vi "Main 硬體參數.vi"() -> ()   [LabVIEW 2015]
uses:
  <vilib>/Utility/miscctls.llb/LVPointTypeDef.ctl
panel:
  in  "切割刀數5":i32=10 min=0 max=10 step=1
  in  "功率5":i32=80 min=3 max=80 step=1
  in  "掃描速度5":i32=1000 min=0 max=10000 step=10
  out "output cluster":T1
  in  "?":T2={"掃描速度"=1000, "功率"=80, "切割刀數"=10, "角度"=10.0, "掃描速度2"=1000, "功率2"=80, "切割刀數2"=10, "角度2"=10.0, "掃描速度3"=1000, "功率3"=80, "切割刀數3"=10, "角度3"=10.0, "掃描速度4"=1000, "功率4"=80, "切割刀數4"=10, "角度4"=10.0, "左/右"=""} {"角度4" min=0.0 max=10.0 step=1.0; "角度3" min=0.0 max=10.0 step=1.0; "角度2" min=0.0 max=10.0 step=1.0; "角度" min=0.0 max=10.0 step=1.0; "切割刀數4" min=0 max=10 step=1; "功率4" min=3 max=80 step=1; "掃描速度4" min=0 max=1000 step=10; "切割刀數3" min=0 max=10 step=1; "功率3" min=3 max=80 step=1; "掃描速度3" min=0 max=1000 step=10; "切割刀數" min=0 max=10 step=1; "功率" min=3 max=80 step=1; "掃描速度" min=0 max=1000 step=10; "切割刀數2" max=10 step=1; "掃描速度2" min=0 max=1000 step=10; "功率2" min=3 max=80 step=1}
  in  "儲存":bool
  in  "離開":bool
  # "硬體參數"
  # "每日點檢"
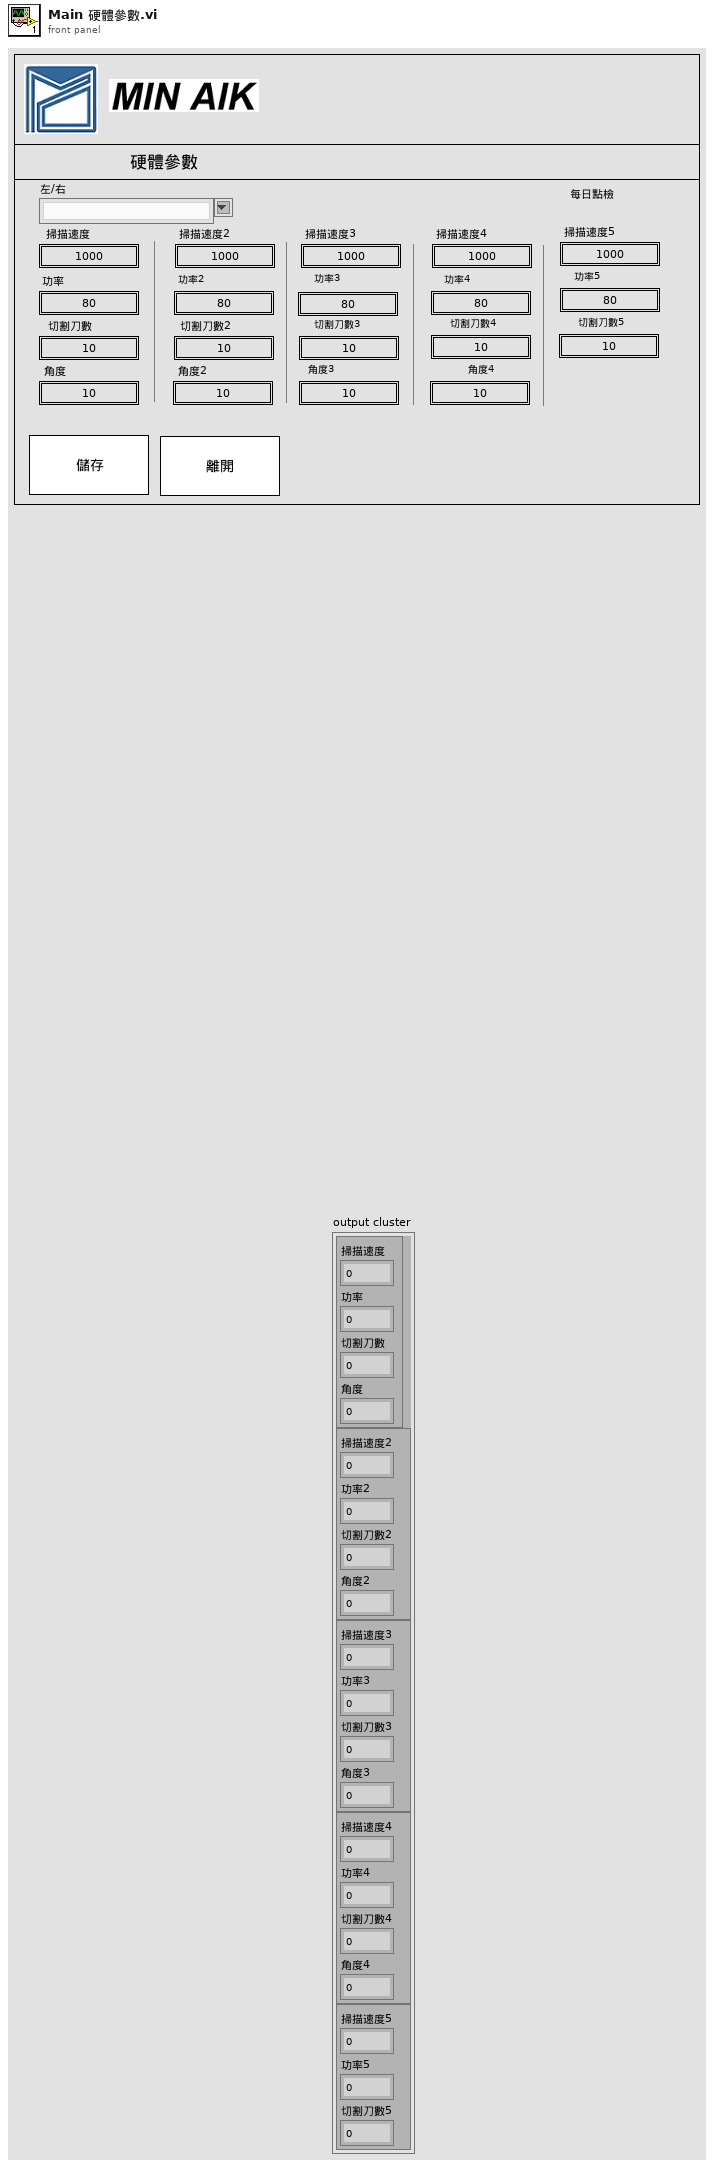
[diagram p1: front panel]
types:
  T1 = cluster{cluster{"掃描速度":i32, "功率":i32, "切割刀數":i32, "角度":dbl}, cluster{"掃描速度2":i32, "功率2":i32, "切割刀數2":i32, "角度2":dbl}, cluster{"掃描速度3":i32, "功率3":i32, "切割刀數3":i32, "角度3":dbl}, cluster{"掃描速度4":i32, "功率4":i32, "切割刀數4":i32, "角度4":dbl}, cluster{"掃描速度5":i32, "功率5":i32, "切割刀數5":i32}}
  T2 = cluster{"掃描速度":i32, "功率":i32, "切割刀數":i32, "角度":dbl, "掃描速度2":i32, "功率2":i32, "切割刀數2":i32, "角度2":dbl, "掃描速度3":i32, "功率3":i32, "切割刀數3":i32, "角度3":dbl, "掃描速度4":i32, "功率4":i32, "切割刀數4":i32, "角度4":dbl, "左/右":string}
  T3 = cluster{"功率":u8, "掃描速率(刀速) ":u16, "雷射半徑":dbl, "刀數":u32}
  T4 = typedef "Action_Data.ctl" = enum16{"Initialize", "Get Data", "Set Data", "Delete Data", "Idle"}
  T5 = typedef "LVPointTypeDef.ctl" = cluster{"Horizontal":i16, "Vertical":i16}
  T6 = cluster{"掃描速度":i32, "功率":i32, "切割刀數":i32, "角度":dbl}
  T7 = cluster{"掃描速度3":i32, "功率3":i32, "切割刀數3":i32, "角度3":dbl}
  T8 = cluster{"掃描速度4":i32, "功率4":i32, "切割刀數3":i32, "角度4":dbl}
  T9 = cluster{"掃描速度2":i32, "功率2":i32, "切割刀數":i32, "角度2":dbl}
  T10 = cluster{cluster{"掃描速度":i32, "功率":i32, "切割刀數":i32, "角度":dbl}, cluster{"掃描速度2":i32, "功率2":i32, "切割刀數":i32, "角度2":dbl}, cluster{"掃描速度3":i32, "功率3":i32, "切割刀數3":i32, "角度3":dbl}, cluster{"掃描速度4":i32, "功率4":i32, "切割刀數3":i32, "角度4":dbl}, cluster{"掃描速率(刀速) ":u16, "功率":u8, "刀數":u32}}
  T11 = cluster{"name or relative path":string, "Variant":variant}
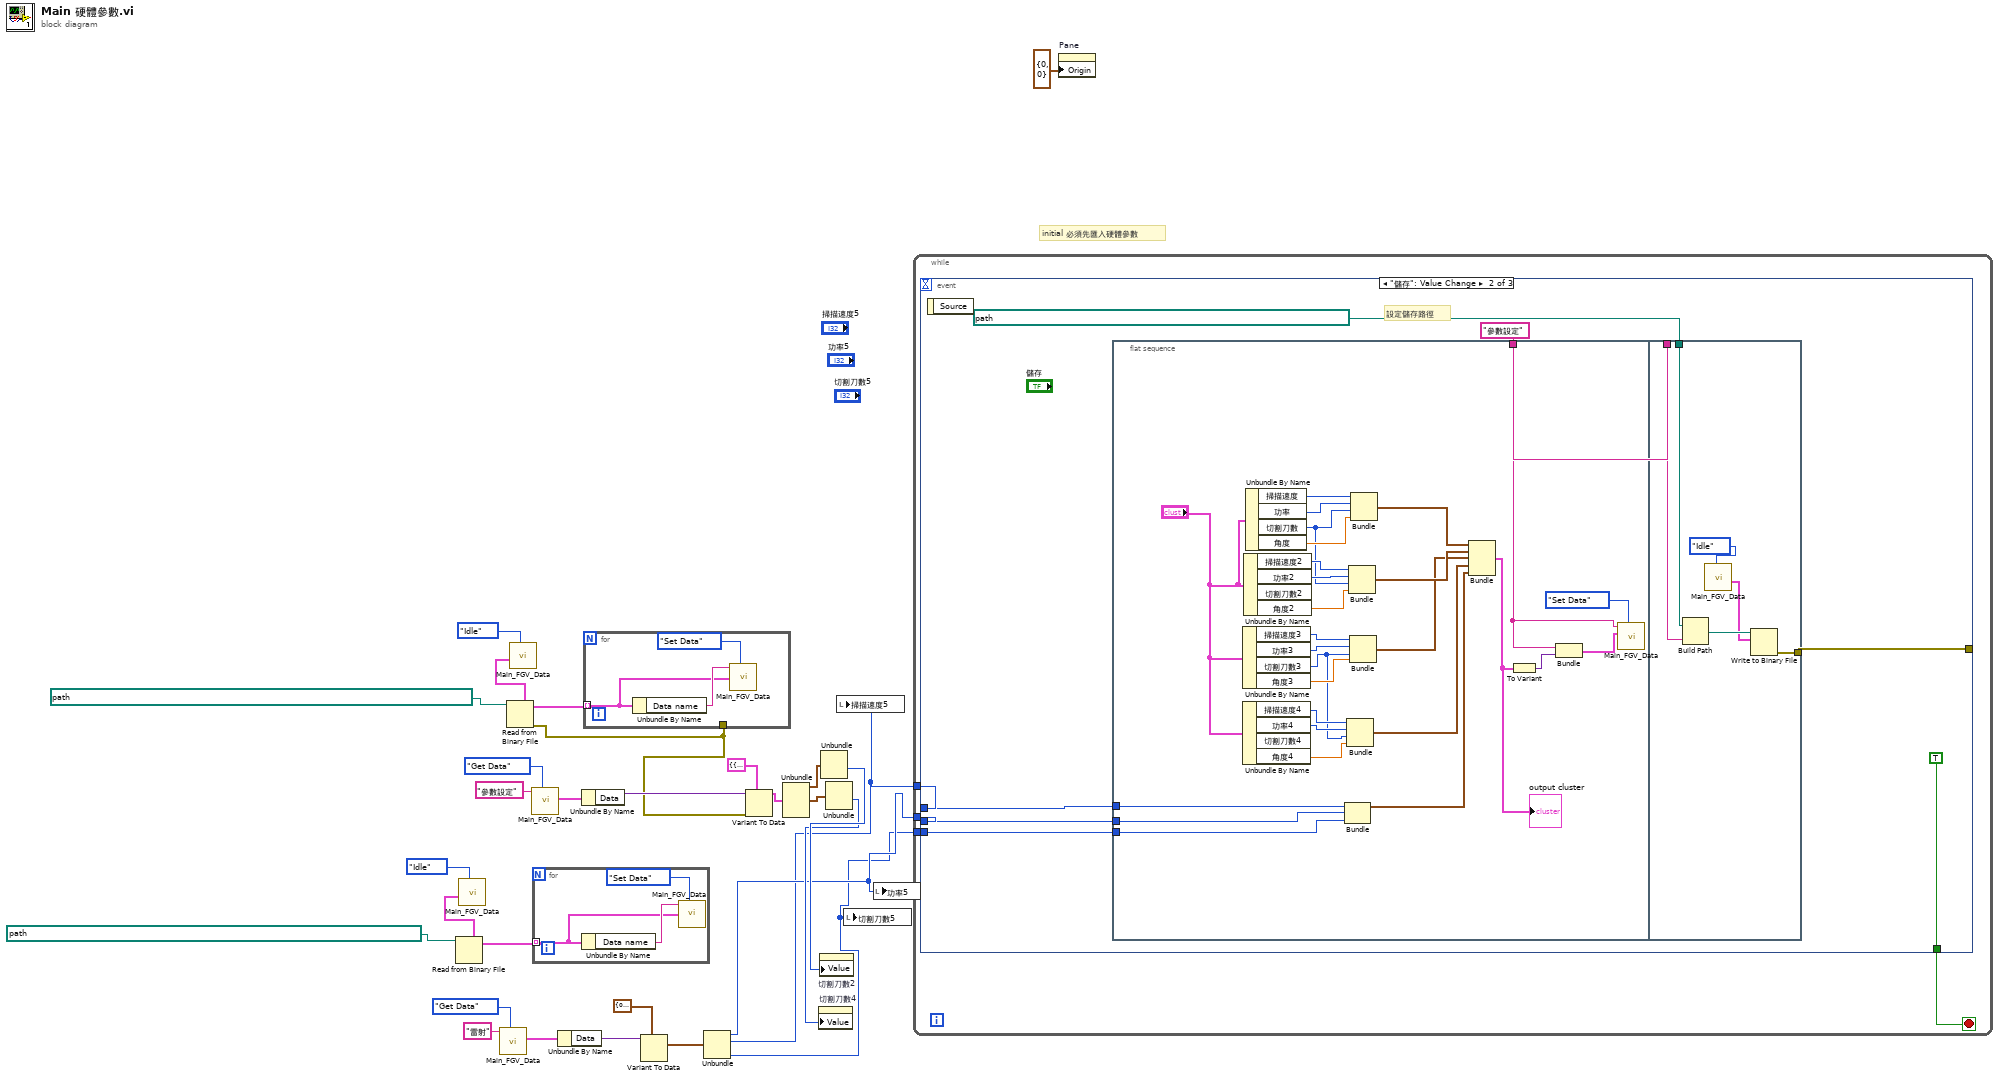
[diagram p0: block diagram]
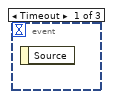
[diagram p2: hidden frame]
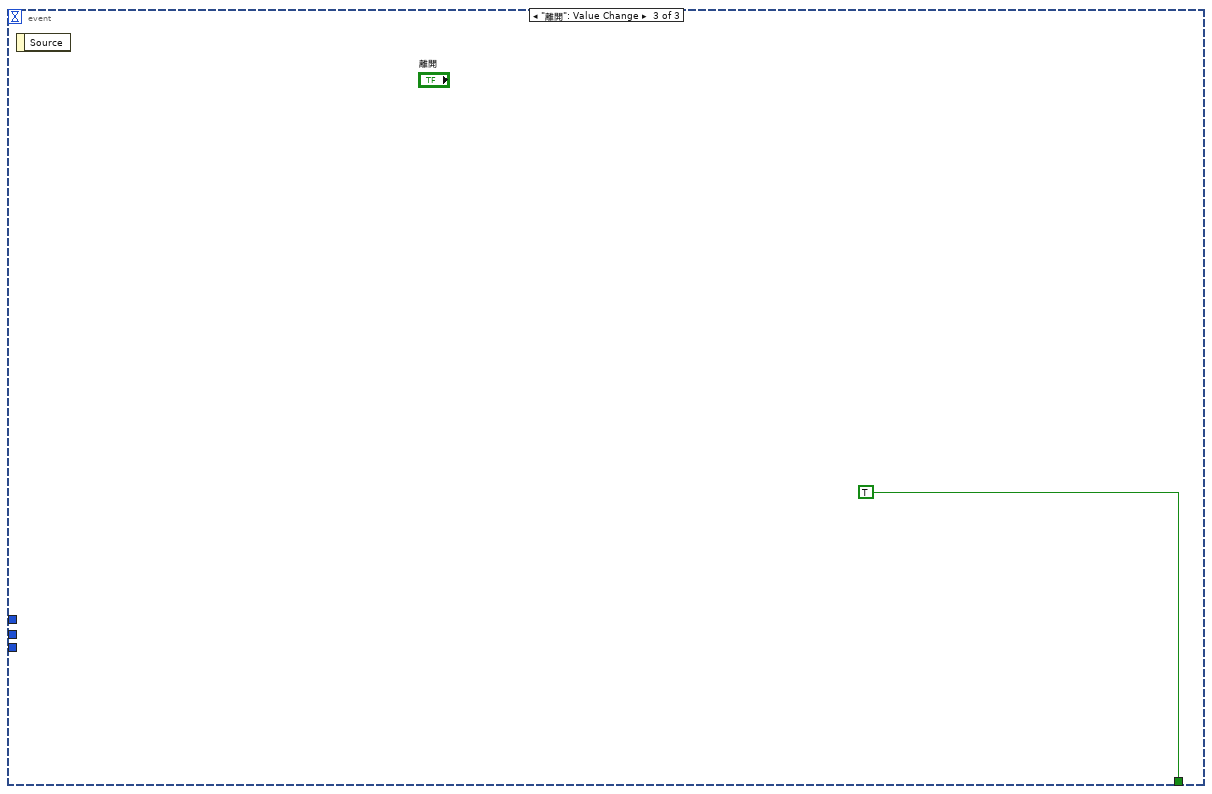
[diagram p3: hidden frame]
diagram:
  # "initial 必須先匯入硬體參數"
  n1 = call "Main_FGV_Data.vi"("Action_Data"=Action_Data."Idle") -> ("Data Array out"=w12:cluster{"Data name":string, "Data":variant}[])  [unwired: 9 in, 1 out]
  n2 = Read from Binary File(5:w12, 11:path "C:/Users/noname/Desktop/Main-Page/四穴雷切/Data資料夾/點檢Data/點檢Data左" ("file (use dialog)")) -> (2:w13:cluster{"Data name":string, "Data":variant}[])  [unwired: 4 in, 3 out]
  n3 = call "Main_FGV_Data.vi"("Action_Data"=Action_Data."Get Data", "Data name"="雷射") -> ("Data  Out"=w7:cluster{"Data name":string, "Data":variant})  [unwired: 8 in, 1 out]
  n4 = call "Main_FGV_Data.vi"("Action_Data"=Action_Data."Idle") -> ("Data Array out"=w23:cluster{"Data name":string, "Data":variant}[])  [unwired: 9 in, 1 out]
  n5 = Read from Binary File(5:w23, 11:path "C:/Users/noname/Desktop/Main-Page/四穴雷切/Data資料夾/參數設定Data/參數設定" ("file (use dialog)")) -> (0:w21:errorcluster, 2:w22:cluster{"Data name":string, "Data":variant}[])  [unwired: 4 in, 2 out]
  n6 = call "Main_FGV_Data.vi"("Action_Data"=Action_Data."Get Data", "Data name"="參數設定") -> ("Data  Out"=w26:cluster{"Data name":string, "Data":variant})  [unwired: 8 in, 1 out]
  n7 = for {
    tunnel: w13 -> [w30] mode=indexing
    n8 = Unbundle By Name(w30) -> ("Data name"=w31:string)
    n9 = call "Main_FGV_Data.vi"("Action_Data"=Action_Data."Set Data", "Data In"=w30, "Data name"=w31) -> ()  [unwired: 7 in, 2 out]
  }
  n10 = Unbundle By Name(w7) -> ("Data"=w6:variant)
  n11 = Unbundle By Name(w26) -> ("Data"=w25:variant)
  n12 = for {
    tunnel: w22 -> [w33] mode=indexing
    tunnel: w21 -> [_]
    n13 = Unbundle By Name(w33) -> ("Data name"=w34:string)
    n14 = call "Main_FGV_Data.vi"("Action_Data"=Action_Data."Set Data", "Data In"=w33, "Data name"=w34) -> ()  [unwired: 7 in, 2 out]
  }
  n15 = Variant To Data(type=T3 {"功率"=0, "掃描速率(刀速) "=0, "雷射半徑"=0.0, "刀數"=0} ("output cluster"), Variant=w6) -> (data=w4:T3)  [unwired: 1 in, 1 out]
  n16 = Unbundle(w4) -> ("功率"=w3:u8, "掃描速率(刀速)"=w2:u16, "刀數"=w1:u32)  [unwired: 1 out]
  n17 = Variant To Data(error in=w21, type=T1 {{"掃描速度"=0, "功率"=0, "切割刀數"=0, "角度"=0.0}, {"掃描速度2"=0, "功率2"=0, "切割刀數2"=0, "角度2"=0.0}, {"掃描速度3"=0, "功率3"=0, "切割刀數3"=0, "角度3"=0.0}, {"掃描速度4"=0, "功率4"=0, "切割刀數4"=0, "角度4"=0.0}, {"掃描速度5"=0, "功率5"=0, "切割刀數5"=0}} ("output cluster"), Variant=w25) -> (data=w20:T1)  [unwired: 1 out]
  n18 = Unbundle(w20) -> (w17:T6, w16:T7)  [unwired: 3 out]
  n19 = Unbundle(w17) -> ("切割刀數"=w18:i32)  [unwired: 3 out]
  n20 = property on="切割刀數2" class="DigNum (strict)"("Value"=w18) -> ()  [unwired: 2 in, 2 out]
  n21 = Unbundle(w16) -> ("切割刀數3"=w15:i32)  [unwired: 3 out]
  n22 = property on="切割刀數4" class="DigNum (strict)"("Value"=w15) -> ()  [unwired: 2 in, 2 out]
  n23 = local write "掃描速度5"(w2) -> ()
  n24 = local write "切割刀數5"(w1) -> ()
  n25 = local write "功率5"(w3) -> ()
  n26 = while {
    tunnel: w1 -> [w38]
    tunnel: w2 -> [w37]
    tunnel: w3 -> [w36]
    stop <- w39 stop-if-true
    n27 = event shown="[1] \"儲存\": Value Change" {
      selector: _ -> [_ _ _]
      dyn-events: _ -> [_ _ _]
      timeout: _ -> [_ _ _]
      tunnel: [_ TRUE TRUE] -> w39
      tunnel: [_ w43 _] -> _
      tunnel: w37 -> [_ w42 _]
      tunnel: w36 -> [_ w41 _]
      tunnel: w38 -> [_ w40 _]
      event Timeout {
        n28 = event-data() -> ()  [unwired: 1 in, 1 out]
      }
      event "儲存": Value Change {
        w44 = "參數設定" ("name or relative path")
        # "設定儲存路徑"
        n29 = event-data() -> ()  [unwired: 1 in, 1 out]
        n30 = flat-sequence {
          tunnel: w44 -> [w65]
          tunnel: w42 -> [w54]
          tunnel: w41 -> [w55]
          tunnel: w40 -> [w56]
          tunnel: path "C:/Users/noname/Desktop/Main-Page/四穴雷切/Data資料夾/參數設定Data" ("file (use dialog) 2") -> [w80]
          tunnel: w44 -> [w79]
          tunnel: [w76] -> w43
          frame #0 {
            n31 = Unbundle By Name("?") -> ("掃描速度3"=w70:i32, "功率3"=w69:i32, "切割刀數3"=w47:i32, "角度3"=w52:dbl)
            n32 = Unbundle By Name("?") -> ("掃描速度4"=w68:i32, "功率4"=w67:i32, "角度4"=w53:dbl)  [unwired: 1 out]
            n33 = Unbundle By Name("?") -> ("掃描速度2"=w72:i32, "功率2"=w71:i32, "角度2"=w51:dbl)  [unwired: 1 out]
            n34 = Unbundle By Name("?") -> ("掃描速度"=w74:i32, "功率"=w73:i32, "切割刀數"=w48:i32, "角度"=w50:dbl)
            n35 = Bundle("掃描速率(刀速)"=w54, "功率"=w55, "刀數"=w56) -> (w58:cluster{"掃描速率(刀速) ":u16, "功率":u8, "刀數":u32})  [unwired: 1 in]
            n36 = Bundle("掃描速度4"=w68, "功率4"=w67, "切割刀數3"=w47, "角度4"=w53) -> (w61:T8)  [unwired: 1 in]
            n37 = Bundle("掃描速度2"=w72, "功率2"=w71, "切割刀數"=w48, "角度2"=w51) -> (w63:T9)  [unwired: 1 in]
            n38 = Bundle("掃描速度3"=w70, "功率3"=w69, "切割刀數3"=w47, "角度3"=w52) -> (w62:T7)  [unwired: 1 in]
            n39 = Bundle("掃描速度"=w74, "功率"=w73, "切割刀數"=w48, "角度"=w50) -> (w64:T6)  [unwired: 1 in]
            n40 = Bundle(w64, w63, w62, w61, w58) -> (w49:T10)  [unwired: 1 in]
            "output cluster" <- w49
            n41 = To Variant(anything=w49) -> (Variant=w60:variant)
            n42 = Bundle("name or relative path"=w65, "Variant"=w60) -> (w59:T11)  [unwired: 1 in]
            n43 = call "Main_FGV_Data.vi"("Action_Data"=Action_Data."Set Data", "Data In"=w59, "Data name"=w65) -> ()  [unwired: 7 in, 2 out]
          }
          frame #1 {
            n44 = Build Path(base path=w80, name or relative path=w79) -> (appended path=w77:path)
            n45 = call "Main_FGV_Data.vi"("Action_Data"=Action_Data."Idle") -> ("Data Array out"=w75:cluster{"Data name":string, "Data":variant}[])  [unwired: 9 in, 1 out]
            n46 = Write to Binary File(file (use dialog)=w77, data=w75) -> (error out=w76:errorcluster)  [unwired: 4 in, 2 out]
          }
        }
      }
      event "離開": Value Change {
        n47 = event-data() -> ()  [unwired: 1 in, 1 out]
      }
    }
  }
  n48 = property on="Pane" class="Pane"("Origin"=T5 {"Horizontal"=0, "Vertical"=0}) -> ()  [unwired: 2 in, 2 out]
